vi "CSM - Debug Console 2.vi"() -> ()   [LabVIEW 2017, in "DebugConsole.lvlib"]
doc: "New version of the CSM Debug Console, you can use this tool:\n1. Select an existing CSM instance, open the front panel and block diagram.\n2. Scan the API interfaces of existing CSM instances.\n3. Select an API interface, call synchronously or asynchronously, view the return value.\n4. View the overall program's running log.\n5. Run Scripts."
uses:
  DebugConsole.lvlib
  _Support/Typedef/_CSM_List Module Scope.ctl
  _Support/GlobalEvent/LogFilter/LogFilter.lvclass/LogFilter.ctl
  _Support/Typedef/_CSM_GlobalLog_MSG.ctl
  _Support/Typedef/_CSM_Response Source Message.ctl
  _Support/Typedef/_CSM_GlobalLog_MSG_TYPE.ctl
  _BroadcastDef.ctl
  AdvanceAPI/CSM - Convert Error to Argument.vi
  _Support/GlobalEvent/GEvt-Generate with Rule Check.vi
  _Support/GlobalEvent/Cache-GEvt Filter Object.vi
  _Support/GlobalEvent/Cache-GEvt Refs.vi
  AdvanceAPI/CSM - Keywords.vi
  _Shared/Trim Single-line Text.vi
  AdvanceAPI/CSM - Make String Arguments Safe.vi
  _Support/GlobalEvent/GEvt-Convert Filter Rules - v1.2.vi
  _Support/ChangeFlag/FlagInstance-GEvt Filter.vi
  _Support/ChangeFlag/FlagInstance-GEvt Refs.vi
  _Support/GlobalEvent/LogFilter/SettingVIs/Set Global CSM Filter.vi
  _Support/GlobalEvent/LogFilter/SettingVIs/Set Global LogType Filter.vi
  _Support/GlobalEvent/LogFilter/SettingVIs/Set Global State Filter.vi
  _Support/GlobalEvent/LogFilter/SettingVIs/Set CSM LogType Filter.vi
  _Support/GlobalEvent/LogFilter/SettingVIs/Set CSM State Filter.vi
  _Support/GlobalEvent/LogFilter/SettingVIs/Set Global StateType Filter.vi
  _Support/GlobalEvent/LogFilter/SettingVIs/Set CSM StateType Filter.vi
  _Support/GlobalEvent/LogFilter/SettingVIs/Set Periodic Log Filter.vi
  _Support/GlobalEvent/LogFilter/SettingVIs/Set CSM Broadcast Filter.vi
  _Support/GlobalEvent/LogFilter/SettingVIs/Set Global Broadcast Filter.vi
  _Support/GlobalEvent/LogFilter/SettingVIs/Set Global UserLog Filter.vi
  _Support/GlobalEvent/LogFilter/SettingVIs/Set CSM UserLog Filter.vi
  _Support/ChangeFlag/ChangeFlag-Read.vi
  _csmHelper/API/Create From VI Reference.vi
  _csmHelper/API/Update lvcsm Section in VI Description.vi
  _csmHelper/API/Destroy.vi
  _csmlite/_PassAllowedMessage - MsgList.vi
  _Support/ChangeFlag/ChangeFlagDB.vi
  _Support/GlobalEvent/FGV-GlobalEventRef(lvlibp).vi
  _Support/GlobalEvent/FGV-GlobalEventQueues(lvlibp).vi
  _Support/GlobalEvent/GEvt-Valid Subscribers.vi
  _Support/GlobalEvent/FGV-GEvt Filter Rules(lvlibp).vi
  _Support/GlobalEvent/LogFilter/LogFilter - Check.vi
  HistoryList.vi
  Script-Window.vi
  Module Information.vi
  _Support/GlobalEvent/LogFilter/LogFilter.lvclass
  Communicable State Machine.lvlib
  _csmHelper/API with lvcsm Support/CSM-Helper API with lvcsm Support.lvlib
  _csmHelper/CSM-Helper.lvclass
  _ui/csm-ui-support.lvlib
  _csmlite/_csmlite.lvlib
  _Shared/CSM Shared.lvlib
  _csmlite/_action.ctl
panel:
  in  "Scope":T1
  in  "Refresh CSMs Button":bool
  in  "CSM":string(combo)
  in  "Write lvcsm in Description":bool
  out "inlvlibp":bool
  in  "RetainWireValues":bool
  in  "Toolbar.Exit":bool
  in  "Toolbar.Open FP":bool
  in  "Toolbar.Open BD":bool
  in  "Refresh lvcsm Cache":bool
  in  "Console":T2(tab)
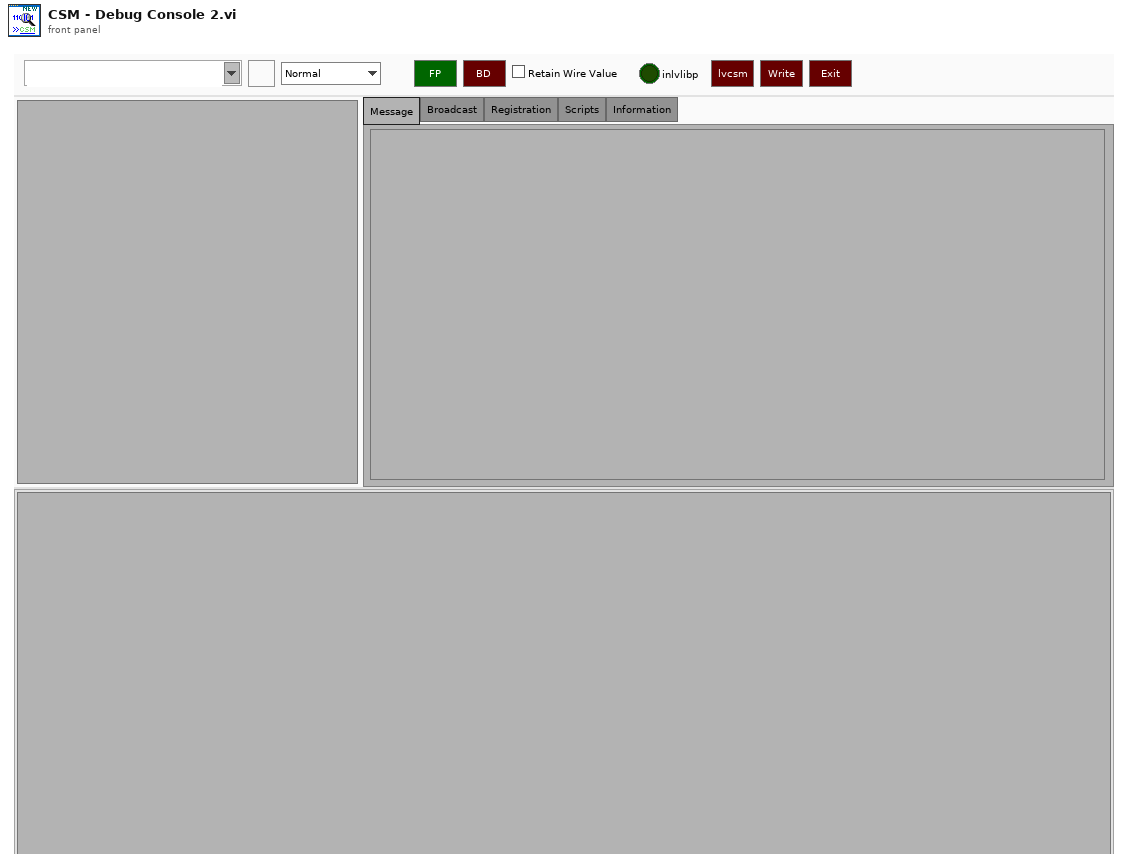
[diagram p1: front panel]
types:
  T1 = typedef "Communicable State Machine.lvlib/_CSM_List Module Scope.ctl" = enum16{"Normal", "System Only", "All"}
  T2 = enum32{"Message", "Broadcast", "Registration", "Scripts", "Information"}
  T3 = cluster{"Left":i32, "Right":i32, "Top":i32, "Bottom":i32}
  T4 = enum32{"Invalid", "Standard", "Closed", "Hidden", "Minimized", "Maximized"}
  T5 = enum32{"invalid app kind", "Development System", "Run Time System", "Student Edition", "Embedded LabVIEW", "Evaluation", "Custom"}
  T6 = typedef "DebugConsole.lvlib/_BroadcastDef.ctl" = enum16{"<no action>", "Macro: Exit", "CSM: Module List Changed", "CSM: Scripts Changed", "CSM: Registration Changed", "CSM: Module Selected", "CSM: Message Excuted", "CSM: Broadcast Excuted", "CSM: Registration Action Excuted", "UI: Try to Change Command"}
  T7 = typedef "_csmlite.lvlib/_action.ctl" = enum16{"Obtain", "Destroy", "Broadcast", "Post", "List"}
  T8 = cluster{"Shift":bool, "Ctrl":bool, "Alt":bool, "Cmd":bool, "Opt":bool}
  T9 = cluster{"Core":cluster{"Current VI Reference":refnum<vi>, "Close Panel on Exit?":bool}, "CSM Global Log Event":refnum<user-event>, "MessageList":string[], "Toobar.advance":refnum<vi>[], "ConsoleUI":refnum<vi>[]}
  T10 = cluster{"Current VI Reference":refnum<vi>, "Close Panel on Exit?":bool}
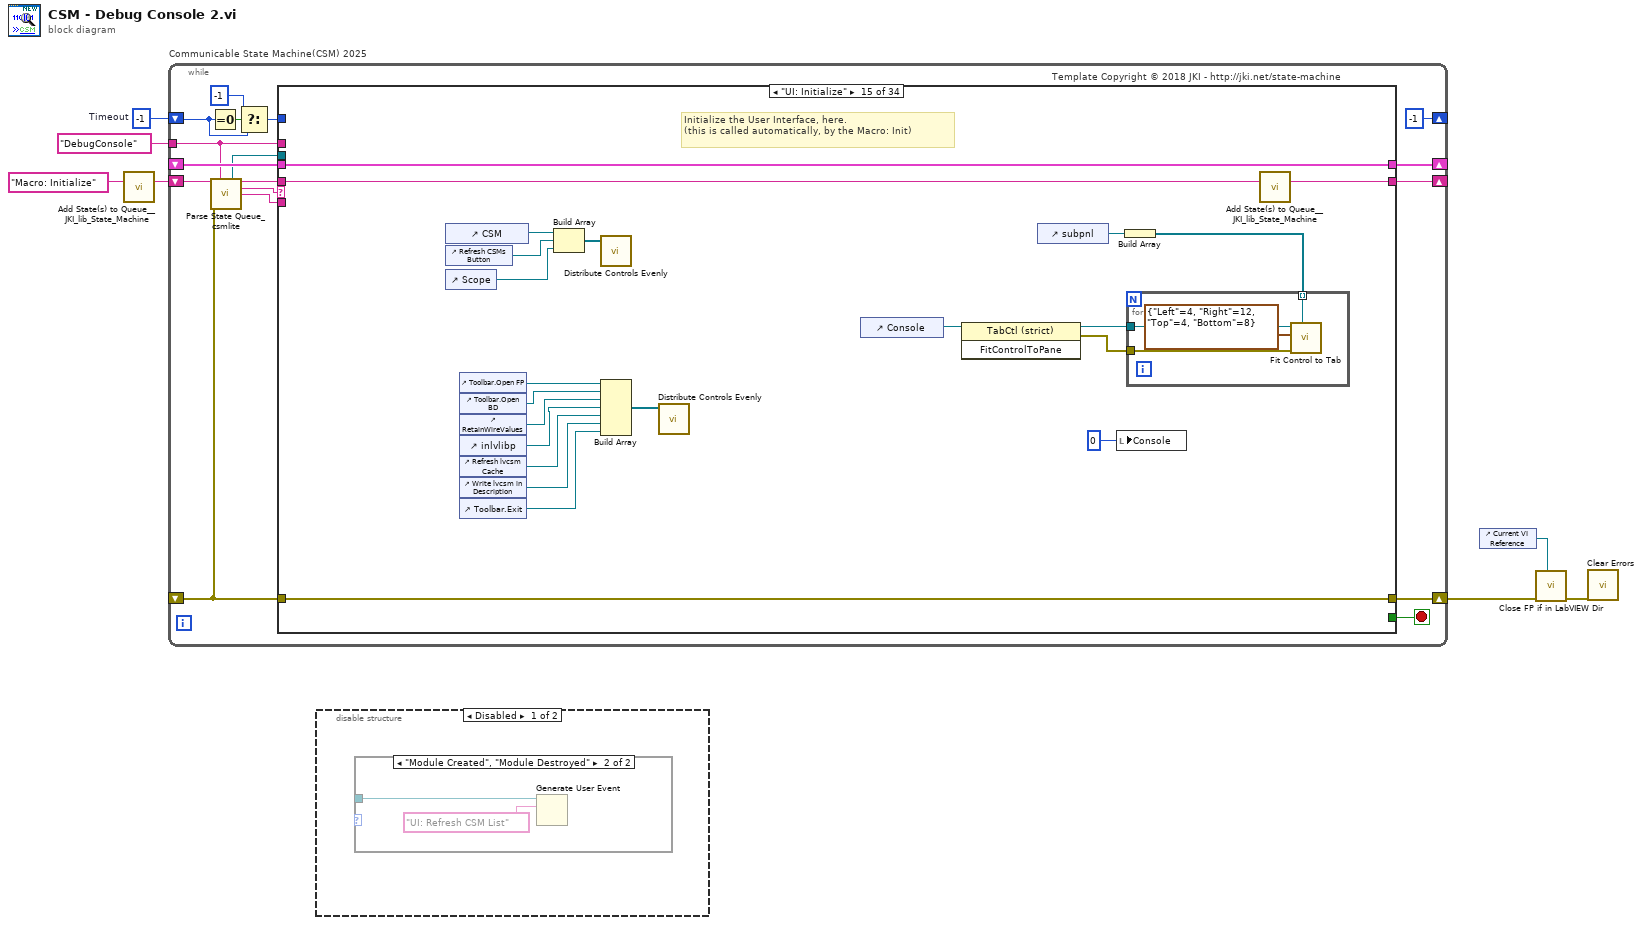
[diagram p0: block diagram]
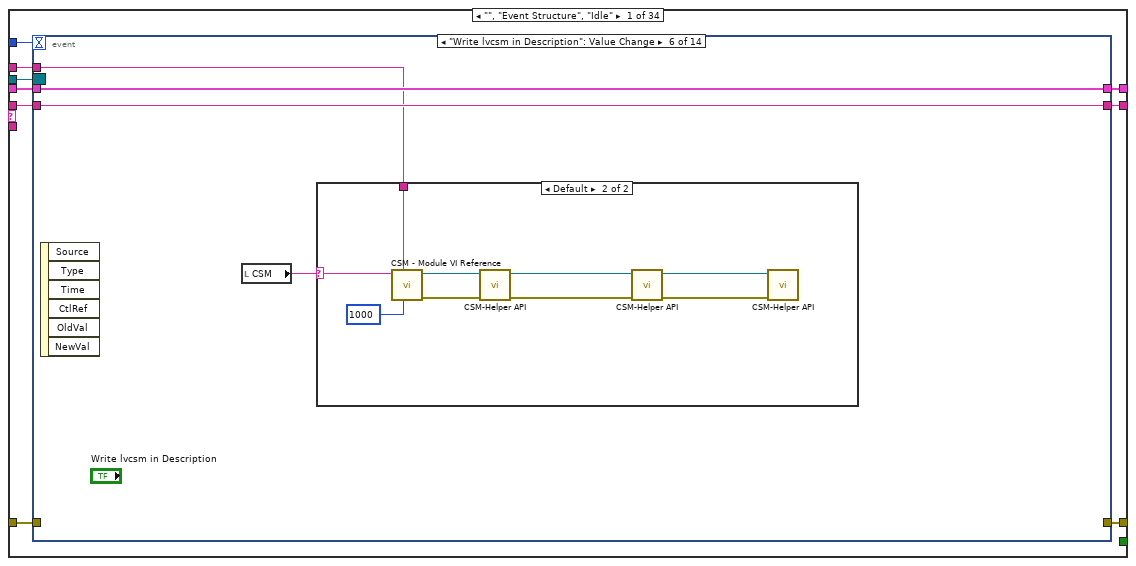
[diagram p4: hidden frame]
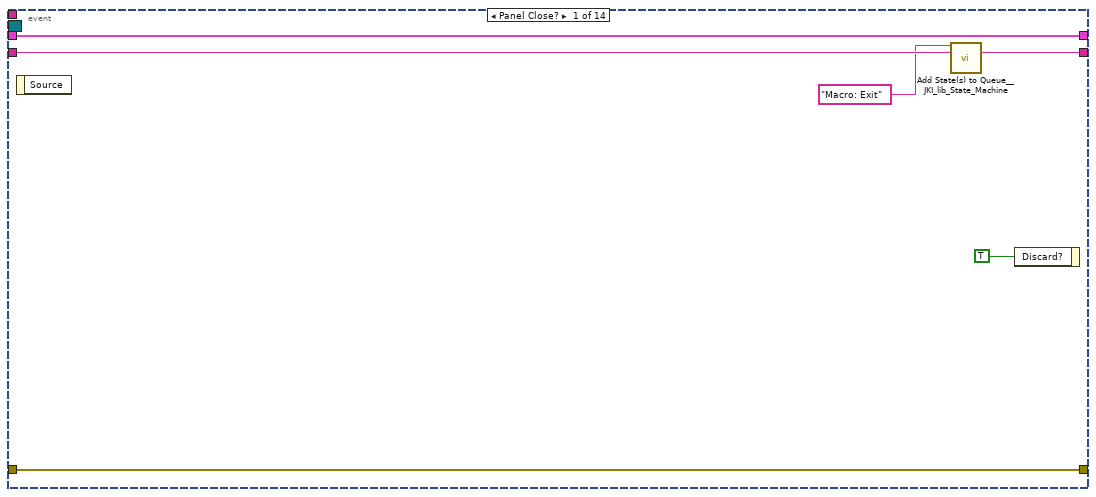
[diagram p5: hidden frame]
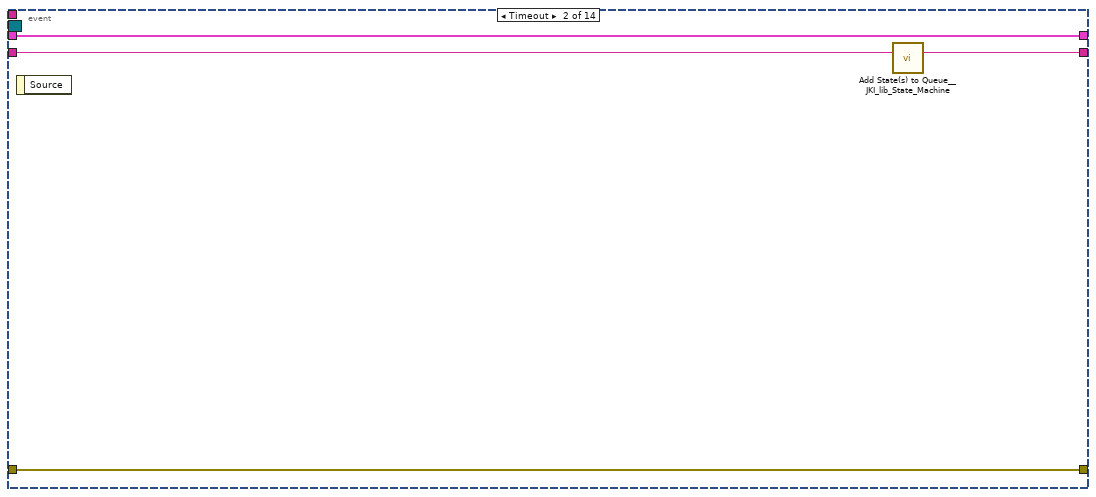
[diagram p6: hidden frame]
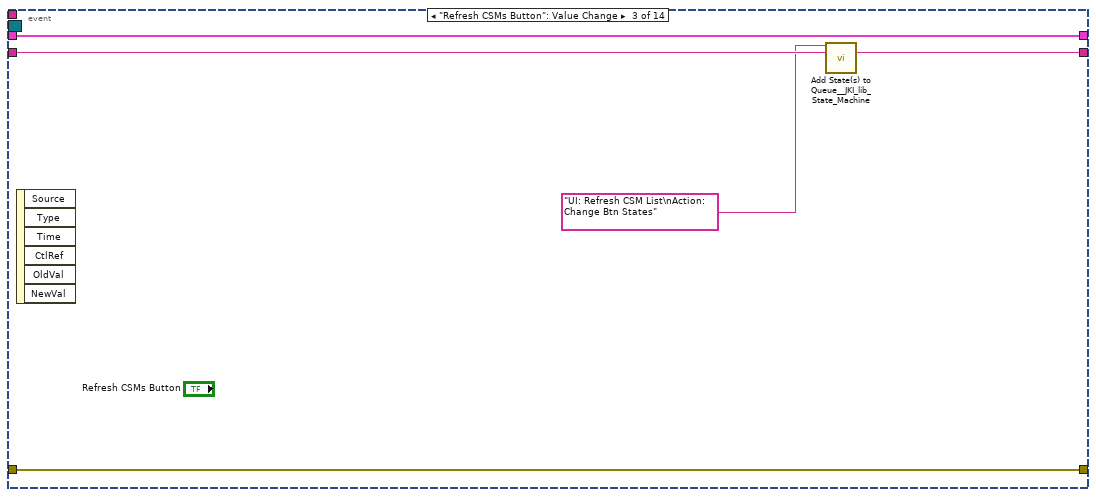
[diagram p7: hidden frame]
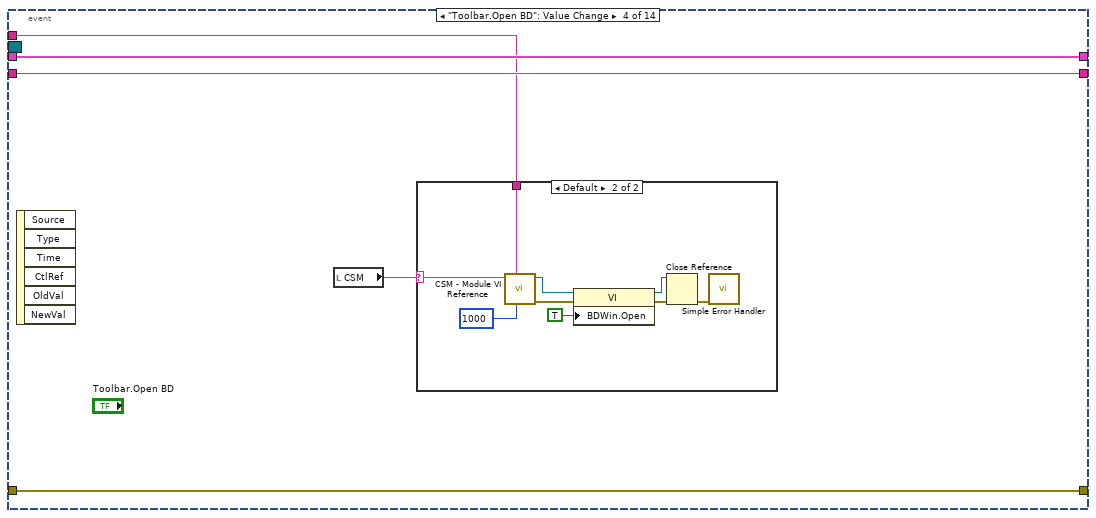
[diagram p8: hidden frame]
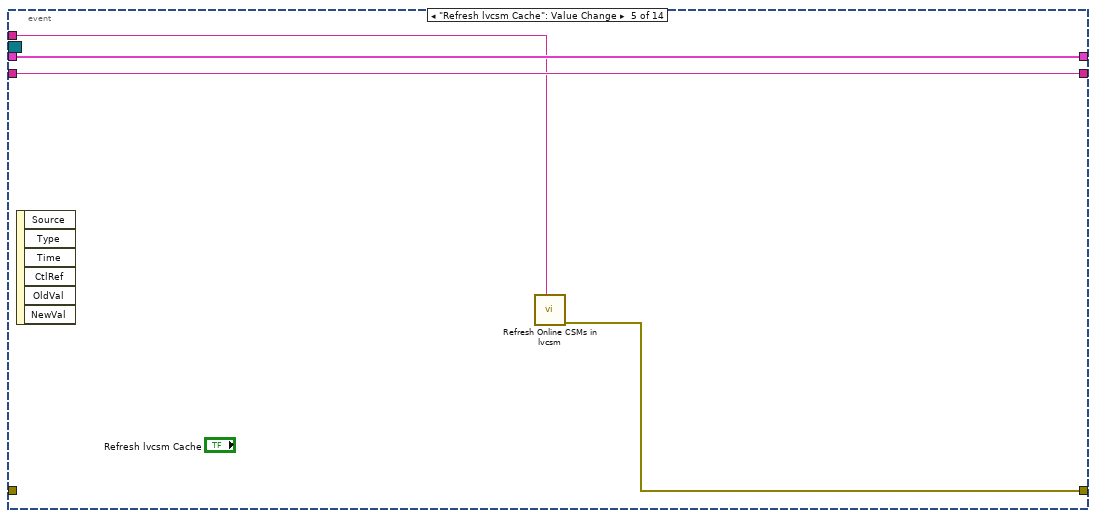
[diagram p10: hidden frame]
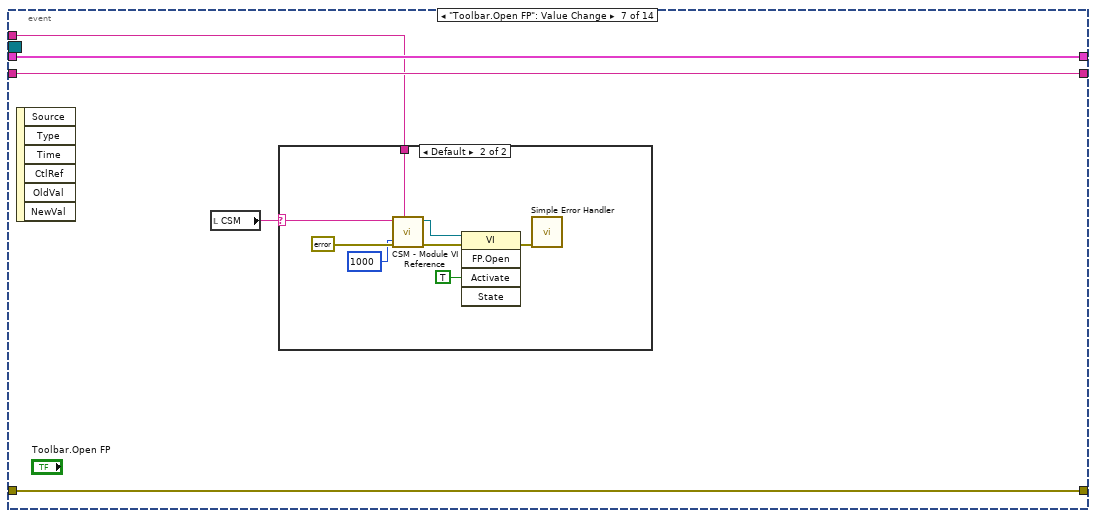
[diagram p12: hidden frame]
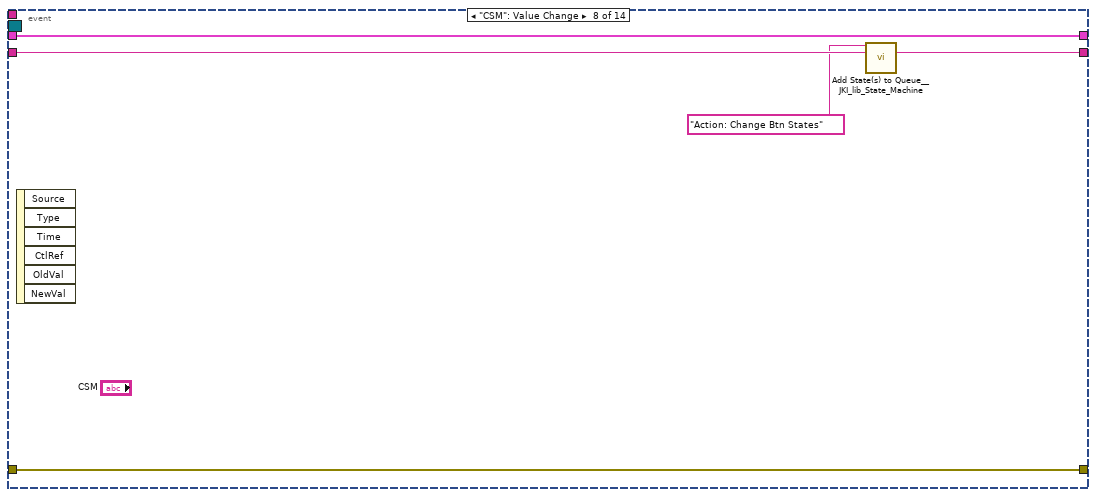
[diagram p14: hidden frame]
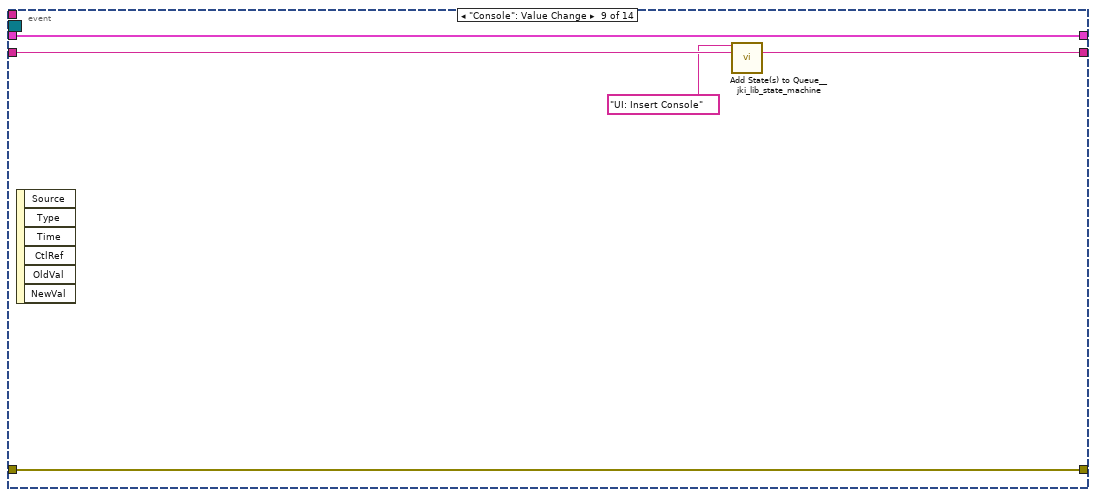
[diagram p15: hidden frame]
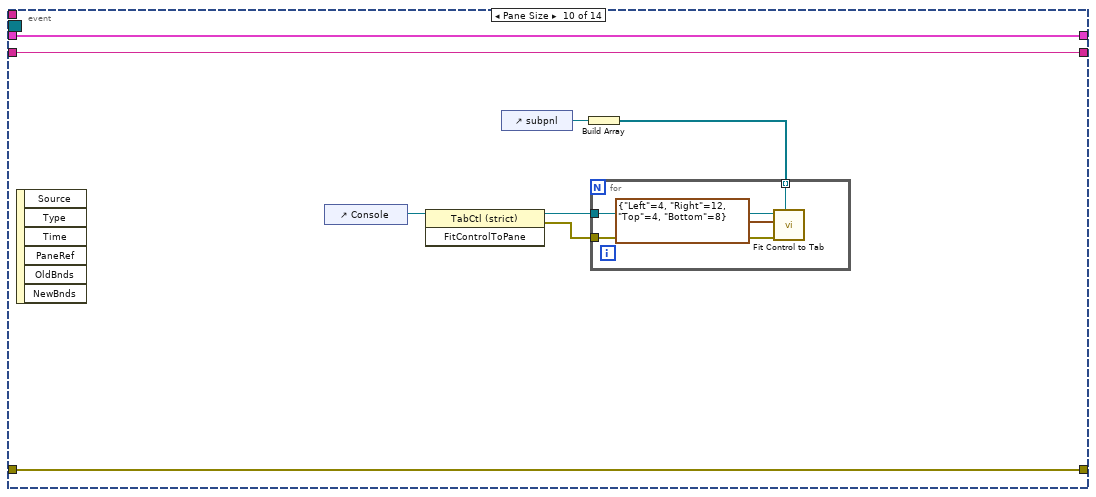
[diagram p16: hidden frame]
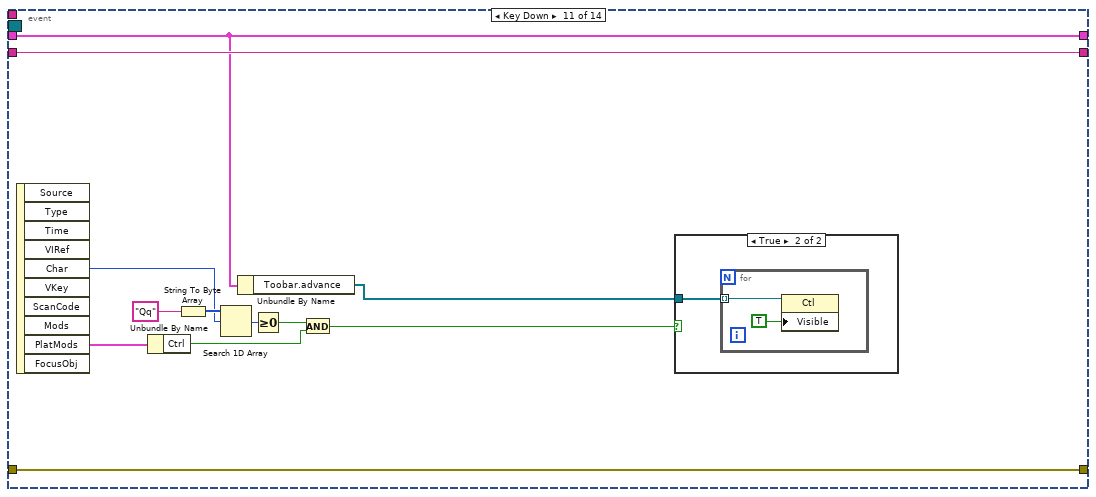
[diagram p17: hidden frame]
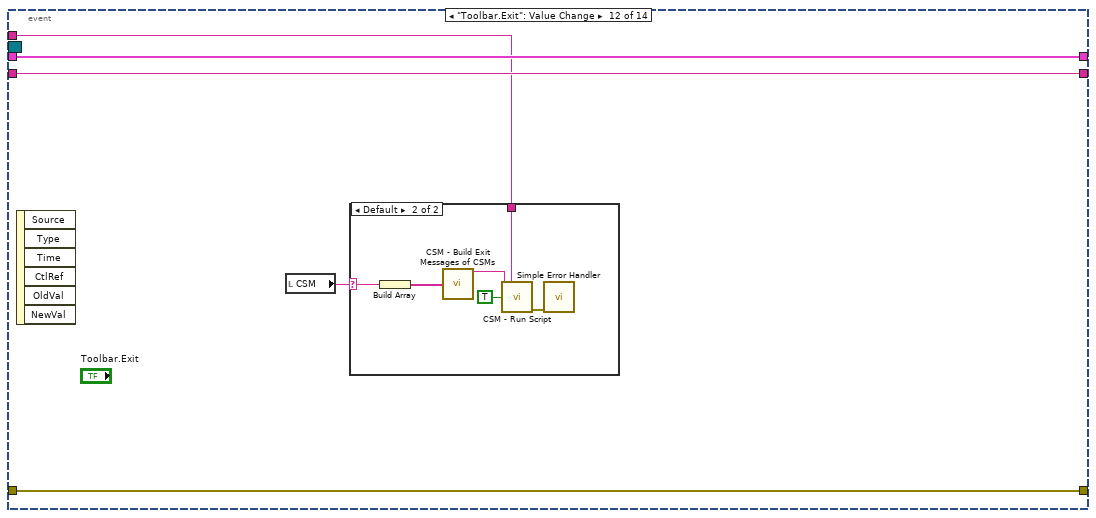
[diagram p19: hidden frame]
diagram:
  w5 = -1  # Timeout
  n1 = call <vilib>:"Add State(s) to Queue__JKI_lib_State_Machine.vi"("State(s) in (\"\")"="Macro: Initialize") -> ("States Out"=w6:string)  [unwired: 14 in]
  n2 = while "Communicable State Machine(CSM) 2025" {
    shift-right: [w17] -> _
    shift-left: _ -> [w16]
    shift-right: [w20] -> w2
    shift-left: _ -> [w15]
    shift-right: [w19] -> _
    shift-left: w6 -> [w21]
    tunnel: "DebugConsole" -> [w9]
    shift-right: [-1 ("Timeout")] -> _
    shift-left: w5 -> [w12]
    stop <- w18 stop-if-true
    # "Template Copyright © 2018 JKI - http://jki.net/state-machine"
    n3 = Equal To 0?(x=w12) -> (x = 0?=w14:bool)
    n4 = call "Parse State Queue_csmlite.vi"("State Queue"=w21, "Current Module(\"\" to generate an ID)"=w9, "Error In (no error)"=w15) -> ("Event Registration Refnum"=w8:refnum<event-registration>, "Remaining States"=w23:string, "Current State"=w24:string, "Arguments"=w22:string)  [unwired: 9 in]
    n5 = Select(t=-1 ("Timeout"), s=w14, f=w12) -> (s? t:f=w11:i32)
    n6 = case shown="\"UI: Initialize\"" w24 {
      selector: w24 -> [_ _ w171 _ _ _ _ _ _ _ _ _ _ _ _ _ _ _ _ _ _ _ _ _ _ _ _ _ _ _ _ _ _ _]
      tunnel: w23 -> [w33 w170 w175 w194 w201 w206 w210 w219 w226 w229 w231 w241 w256 w260 w282 w292 w303 w380 w397 w417 w433 w440 w443 w448 w453 w464 w485 w491 w510 w515 w534 w553 w572 w591]
      tunnel: w22 -> [_ _ _ _ _ _ _ _ _ _ _ w237 _ _ _ w287 w297 _ w394 _ _ _ _ _ _ _ _ _ _ _ _ _ _ _]
      tunnel: w16 -> [w31 w167 w173 w187 w198 w204 w207 _ w225 w228 w230 w239 w251 w257 w279 w290 w299 w379 w396 w416 w432 w438 w442 w445 w450 w461 w482 w490 w509 w514 w533 w552 w571 w590]
      tunnel: [w30 w168 w177 w191 errorcluster {"status"=FALSE, "code"=0, "source"=""} ("error out") w203 w208 w216 w227 _ _ w240 w252 w258 w280 w288 w300 w381 w398 w418 w434 w441 w444 w446 w451 w462 w483 w492 w511 w516 w535 w554 w573 w592] -> w20
      tunnel: w15 -> [w29 w168 w176 w191 w197 w203 w208 w216 w227 _ _ w240 w253 w258 w280 w289 w301 w381 w398 w418 w434 w441 w444 w446 w451 w462 w483 w492 w511 w516 w535 w554 w573 w592]
      tunnel: [w32 w169 w174 w193 w200 w205 w209 w218 w226 w229 w231 w241 w255 w259 w281 w291 w302 w380 w397 w417 w433 w440 w443 w447 w452 w463 w484 w491 w510 w515 w534 w553 w572 w591] -> w19
      tunnel: [_ _ _ _ _ TRUE _ _ _ _ _ _ _ _ _ _ _ _ _ _ _ _ _ _ _ _ _ _ _ _ _ _ _ _] -> w18
      tunnel: [w28 w167 w173 w192 w198 w204 w207 w217 w222 w228 w230 w233 w251 w257 w279 w290 w299 w379 w396 w416 w432 w438 w442 w445 w450 w461 w482 w490 w509 w513 w532 w551 w570 w589] -> w17
      tunnel: w11 -> [w27 _ _ _ _ _ _ _ _ _ _ _ _ _ _ _ _ _ _ _ _ _ _ _ _ _ _ _ _ _ _ _ _ _]
      tunnel: w9 -> [w26 _ _ _ w195 _ _ _ _ _ _ _ _ _ _ _ _ _ _ w405 w421 _ _ _ _ w454 _ w488 w507 w512 w531 w550 w569 w588]
      tunnel: w8 -> [w25 _ _ _ _ _ _ _ _ _ _ _ _ _ _ _ _ _ _ _ _ _ _ _ _ _ _ _ _ _ _ _ _ _]
      frame "", "Event Structure", "Idle" {
        n7 = event shown="[5] \"Write lvcsm in Description\": Value Change" {
          selector: w25 -> [_ _ _ _ _ _ _ _ _ _ _ _ _ _]
          dyn-events: _ -> [_ _ _ _ _ _ _ _ _ _ _ _ _ _]
          timeout: w27 -> [_ _ _ _ _ _ _ _ _ _ _ _ _ _]
          tunnel: w33 -> [w39 w43 w46 w53 w66 w70 w84 w94 w99 w110 w126 w134 w148 w163]
          tunnel: [w38 w42 w45 w53 w66 w70 w84 w95 w100 w110 w126 w134 w148 w164] -> w32
          tunnel: w31 -> [w36 w40 w47 w52 w65 w69 w83 w96 w101 w108 w115 w133 w146 w165]
          tunnel: [w37 w41 w48 w50 w63 _ w81 w97 w102 w109 w125 w132 w147 w166] -> w30
          tunnel: w29 -> [w37 w41 w48 w50 _ _ w81 w97 w102 w109 w125 w132 w147 w166]
          tunnel: [w36 w40 w47 w52 w65 w69 w83 w96 w101 w108 w115 w133 w146 w165] -> w28
          tunnel: w26 -> [_ _ _ w49 w64 w67 w80 _ _ _ _ w130 w144 _]
          event Panel Close? {
            n8 = event-data() -> ()  [unwired: 1 in, 1 out]
            n9 = call <vilib>:"Add State(s) to Queue__JKI_lib_State_Machine.vi"("State(s) in Front (\"\")"="Macro: Exit", "State(s) in (\"\")"=w39) -> ("States Out"=w38:string)  [unwired: 13 in]
            n10 = event-data("Discard?"=TRUE) -> ()  [unwired: 1 in, 1 out]
          }
          event Timeout {
            n11 = event-data() -> ()  [unwired: 1 in, 1 out]
            n12 = call <vilib>:"Add State(s) to Queue__JKI_lib_State_Machine.vi"("State(s) in (\"\")"=w43) -> ("States Out"=w42:string)  [unwired: 14 in]
          }
          event "Refresh CSMs Button": Value Change {
            n13 = event-data() -> ()  [unwired: 1 in, 6 out]
            n14 = call <vilib>:"Add State(s) to Queue__JKI_lib_State_Machine.vi"("State(s) in Front (\"\")"="UI: Refresh CSM List\nAction: Change Btn States" ("State(s) in Front (\"\")"), "State(s) in (\"\")"=w46) -> ("States Out"=w45:string)  [unwired: 13 in]
          }
          event "Toolbar.Open BD": Value Change {
            n15 = event-data() -> ()  [unwired: 1 in, 6 out]
            n16 = local read "CSM"() -> (w51:string)
            n17 = case shown="Default" w51 {
              selector: w51 -> [_ w61]
              tunnel: w49 -> [_ w60]
              frame "" {
              }
              frame Default {
                n18 = call "CSM - Module VI Reference.vi"("Response Timeout (-2 Using Global Settings)"=1000 ("Response Timeout(5000 ms)"), "Current Module (\"\" to Generate an ID)"=w60, "CSM Name"=w61) -> ("error out"=w54:errorcluster, "CSM Module VIRef"=w59:refnum<vi>)  [unwired: 7 in]
                n19 = property class="VI"(reference=w59, error in=w54, "BDWin.Open"=TRUE ("Block Diagram Window:Open")) -> (reference out=w57:refnum<vi>, error out=w56:errorcluster)
                n20 = Close Reference(reference=w57, error in (no error)=w56) -> (error out=w62:errorcluster)
                n21 = call <vilib>:"Simple Error Handler.vi"("error in (no error)"=w62) -> ()  [unwired: 4 in, 5 out]
              }
            }
          }
          event "Refresh lvcsm Cache": Value Change {
            n22 = event-data() -> ()  [unwired: 1 in, 6 out]
            n23 = call "Refresh Online CSMs in lvcsm.vi"("Caller"=w64) -> ("error out"=w63:errorcluster)  [unwired: 9 in, 1 out]
          }
          event "Write lvcsm in Description": Value Change {
            n24 = event-data() -> ()  [unwired: 1 in, 6 out]
            n25 = local read "CSM"() -> (w68:string)
            n26 = case shown="Default" w68 {
              selector: w68 -> [_ w75]
              tunnel: w67 -> [_ w71]
              frame "" {
              }
              frame Default {
                n27 = call "CSM - Module VI Reference.vi"("Response Timeout (-2 Using Global Settings)"=1000 ("Response Timeout(5000 ms)"), "Current Module (\"\" to Generate an ID)"=w71, "CSM Name"=w75) -> ("error out"=w73:errorcluster, "CSM Module VIRef"=w72:refnum<vi>)  [unwired: 7 in]
                n28 = call-poly "CSM-Helper API.vi"("error in (no error)"=w73, "VI"=w72) -> ("error out"=w79:errorcluster, "CSM-Helper.lvclass"=w78:refnum<class "CSM-Helper.lvclass">)  [unwired: 8 in]
                n29 = call-poly "CSM-Helper API.vi"("error in (no error)"=w79, "CSM-Helper in"=w78) -> ("error out"=w77:errorcluster, "CSM-Helper out"=w76:refnum<class "CSM-Helper.lvclass">)  [unwired: 8 in]
                n30 = call-poly "CSM-Helper API.vi"("error in (no error)"=w77, "CSM-Helper in"=w76) -> ()  [unwired: 8 in, 2 out]
              }
            }
          }
          event "Toolbar.Open FP": Value Change {
            n31 = event-data() -> ()  [unwired: 1 in, 6 out]
            n32 = local read "CSM"() -> (w82:string)
            n33 = case shown="Default" w82 {
              selector: w82 -> [_ w92]
              tunnel: w80 -> [_ w90]
              frame "" {
              }
              frame Default {
                n34 = call "CSM - Module VI Reference.vi"("Response Timeout (-2 Using Global Settings)"=1000 ("Response Timeout(5000 ms)"), "Current Module (\"\" to Generate an ID)"=w90, "error in (no error)"=errorcluster {"status"=FALSE, "code"=0, "source"=""}, "CSM Name"=w92) -> ("error out"=w86:errorcluster, "CSM Module VIRef"=w87:refnum<vi>)  [unwired: 6 in]
                n35 = invoke on="Invoke Node" class="VI" method="FP.Open"(reference=w87, error in=w86, "Activate"=TRUE ("Activate?")) -> (error out=w91:errorcluster)  [unwired: 2 in, 4 out]
                n36 = call <vilib>:"Simple Error Handler.vi"("error in (no error)"=w91) -> ()  [unwired: 4 in, 5 out]
              }
            }
          }
          event "CSM": Value Change {
            n37 = event-data() -> ()  [unwired: 1 in, 6 out]
            n38 = call <vilib>:"Add State(s) to Queue__JKI_lib_State_Machine.vi"("State(s) in Front (\"\")"="Action: Change Btn States" ("State(s) in Front (\"\")"), "State(s) in (\"\")"=w94) -> ("States Out"=w95:string)  [unwired: 13 in]
          }
          event "Console": Value Change {
            n39 = event-data() -> ()  [unwired: 1 in, 6 out]
            n40 = call <vilib>:"Add State(s) to Queue__jki_lib_state_machine.vi"("State(s) in Front (\"\")"="UI: Insert Console" ("State(s) in Front (\"\")"), "State(s) in (\"\")"=w99) -> ("States Out"=w100:string)  [unwired: 13 in]
          }
          event Pane Size {
            n41 = event-data() -> ()  [unwired: 1 in, 6 out]
            n42 = control-ref of="Console"() -> (w105:refnum<vi>)
            n43 = invoke class="TabCtl (strict)" method="FitControlToPane"(reference=w105) -> (reference out=w107:refnum<vi>, error out=w106:errorcluster)  [unwired: 2 in, 1 out]
            n44 = control-ref of="subpnl"() -> (w104:refnum<vi>)
            n45 = Build Array(w104) -> (w103:refnum<vi>[])
            n46 = for {
              tunnel: w107 -> [w114]
              tunnel: w103 -> [w113] mode=indexing
              tunnel: w106 -> [w112]
              n47 = call "Fit Control to Tab.vi"("Control"=w113, "error in (no error)"=w112, "Margin"=T3 {"Left"=4, "Right"=12, "Top"=4, "Bottom"=8}, "TabRef"=w114) -> ()  [unwired: 3 in, 3 out]
            }
          }
          event Key Down {
            n48 = event-data() -> ("Char"=w116:i16, "PlatMods"=w117:T8)  [unwired: 1 in, 8 out]
            n49 = Unbundle By Name(w117) -> ("Ctrl"=w120:bool)
            n50 = String To Byte Array(string="Qq") -> (unsigned byte array=w122:u8[])
            n51 = Search 1D Array(1D array=w122, element=w116) -> (index of element=w123:i32)  [unwired: 1 in]
            n52 = Unbundle By Name(w115) -> ("Toobar.advance"=w118:refnum<vi>[])
            n53 = Greater Or Equal To 0?(x=w123) -> (x >= 0?=w124:bool)
            n54 = And(x=w124, y=w120) -> (x .and. y?=w119:bool)
            n55 = case shown="True" w119 {
              tunnel: w118 -> [_ w127]
              frame False {
              }
              frame True {
                n56 = for {
                  tunnel: w127 -> [w129] mode=indexing
                  n57 = property class="Ctl"(reference=w129, "Visible"=TRUE) -> ()  [unwired: 1 in, 2 out]
                }
              }
            }
          }
          event "Toolbar.Exit": Value Change {
            n58 = event-data() -> ()  [unwired: 1 in, 6 out]
            n59 = local read "CSM"() -> (w131:string)
            n60 = case shown="Default" w131 {
              selector: w131 -> [_ w137]
              tunnel: w130 -> [_ w140]
              frame "" {
              }
              frame Default {
                n61 = Build Array(w137) -> (w136:string[])
                n62 = call "CSM - Build Exit Messages of CSMs.vi"("CSMs"=w136) -> ("States"=w138:string)  [unwired: 14 in]
                n63 = call "CSM - Run Script.vi"("CSM Scripts"=w138, "Current Module (\"\" to Generate an ID)"=w140, "Continue If Error? (F)"=TRUE) -> ("error out"=w139:errorcluster)  [unwired: 10 in, 2 out]
                n64 = call <vilib>:"Simple Error Handler.vi"("error in (no error)"=w139) -> ()  [unwired: 4 in, 5 out]
              }
            }
          }
          event "RetainWireValues": Value Change {
            n65 = event-data() -> ("CtlRef"=w142:refnum<vi>, "OldVal"=w141:bool, "NewVal"=w143:bool)  [unwired: 1 in, 3 out]
            n66 = local read "CSM"() -> (w145:string)
            n67 = case shown="Default" w145 {
              selector: w145 -> [_ w154]
              tunnel: w144 -> [_ w153]
              tunnel: w143 -> [_ w152]
              tunnel: w142 -> [_ w150]
              tunnel: w141 -> [_ w149]
              frame "" {
              }
              frame Default {
                n68 = call "CSM - Module VI Reference.vi"("Current Module (\"\" to Generate an ID)"=w153, "CSM Name"=w154) -> ("error out"=w156:errorcluster, "CSM Module VIRef"=w155:refnum<vi>)  [unwired: 8 in]
                n69 = property class="VI"(reference=w155, error in=w156, "Exec.PostExecutionProbes"=w152) -> (error out=w151:errorcluster)  [unwired: 1 out]
                n70 = case shown="Error" w151 {
                  selector: w151 -> [_ w157]
                  tunnel: w150 -> [_ w159]
                  tunnel: w149 -> [_ w158]
                  frame No Error {
                  }
                  frame Error {
                    n71 = call <vilib>:"Simple Error Handler.vi"("error in (no error)"=w157) -> ()  [unwired: 4 in, 5 out]
                    n72 = property class="Bool (strict)"(reference=w159, "Value"=w158) -> ()  [unwired: 1 in, 2 out]
                  }
                }
              }
            }
          }
          event User Event {
            n73 = event-data() -> ("Message Event"=w162:string)  [unwired: 1 in]
            n74 = call-poly "Pass Allowed Message.vi"("Allowed Message"=string[] ["Macro: Exit", "CSM: Module List Changed", "UI: Try to Change Command"], "JKISM External Event"=w162) -> ("States"=w161:string)  [unwired: 7 in]
            n75 = call <vilib>:"Add State(s) to Queue__JKI_lib_State_Machine.vi"("State(s) in Front (\"\")"=w161, "State(s) in (\"\")"=w163) -> ("States Out"=w164:string)  [unwired: 13 in]
          }
        }
      }
      frame "---------- Core ----------" {
        # "Do not put any code in this frame.\n(it is a separator no-op)"
        n76 = call <vilib>:"Add State(s) to Queue__JKI_lib_State_Machine.vi"("State(s) in (\"\")"=w170) -> ("States Out"=w169:string)  [unwired: 14 in]
      }
      frame Default {
        w180 = 42 items=["No error", "Argument error", "Memory is full", "Out of zone", "End of file", "File already open", "Generic file I/O error", "File not found", "File permission error", "Disk is full", "Duplicate path", "Too many files open", "System feature not enabled", "Resource file not found", "Cannot add resource", "Resource not found", "Image not found", "Image memory error", "Pen does not exist", "Config type invalid", "Config token not found", "Config parse error", "Config memory error", "Bad external code format", "Bad external code offset", "External code not present", "Null window", "Destroy window error", "Null menu", "Print aborted", "Bad print record", "Print driver error", "Windows error during printing", "Memory error during printing", "Print dialog error", "Generic print error", "Invalid device refnum", "Device not found", "Device parameter error", "Device unit error", "Cannot open device", "Device call aborted", "Generic error", "Cancelled by user", "Object ID too low", "Object ID too high", "Object not in heap", "Unknown heap", "Unknown object (invalid DefProc)", "Unknown object (DefProc not in table)", "Message out of range", "Invalid (null) method", "Unknown message", "Manager call not supported", "Bad address", "Network operation in progress", "Network operation timed out", "Connection is busy", "Network attribute not supported", "Network error", "Address in use", "System out of memory", "Connection aborted", "Connection refused", "Not connected", "Already connected", "Connection closed", "Initialization error (interapplication manager)", "Bad occurrence", "Wait on unbound occurrence handler", "Occurrence queue overflow", "Datalog type conflict", "Unused", "Unrecognized type (interapplication manager)", "Memory corrupt", "Failed to make temporary DLL", "Old CIN version", "Drag socket not found", "Failed to load drop-object", "Failed to register OLE object", "Failed to release OLE object", "Format specifier type mismatch", "Unknown format specifier", "Too few format specifiers", "Too many format specifiers", "Scan failed", "Newer CIN version", "Error converting to variant", "Runtime menu error", "Password tampered", "Variant attribute not found", "Incompatible variant data type", "Event data is not available", "Event Store is not present", "Occurrence is not found", "Event Queue is not created", "Event info is not available", "Refnum passed is NULL", "Error retrieving Class GUID", "Error retrieving CoClass GUID", "Error retrieving TypeLib GUID.", "Bad built application magic bytes.", "Specific driver is different from the specific driver associated with the Logical Name.", "There is no session opened to the class driver.", "Max Error", "MAX - Error with config objects", "MAX - Error loading configuration", "MAX - Group not supported"]
        # "Current State"
        # "Do not delete, rename, or modify this frame.\n(this is used to capture unhandled states and typos)"
        # "Handle mistyped state name (developer tool)"
        n77 = Format Into String(format string="Software Exception: Unhandled State \"%s\"." ("message"), error in=w176, w171) -> (resulting string=w179:string, error out=w178:errorcluster)  [unwired: 1 in]
        n78 = call <vilib>:"Error Cluster From Error Code.vi"("show call chain? (False)"=TRUE, "error in (no error)"=w178, "error message (\"\")"=w179, "error code (0)"=w180) -> ("error out"=w177:errorcluster)  [unwired: 5 in]
        n79 = call <vilib>:"Add State(s) to Queue__JKI_lib_State_Machine.vi"("State(s) in (\"\")"=w175) -> ("States Out"=w174:string)  [unwired: 14 in]
      }
      frame "Initialize Core Data" {
        # "Do not delete, rename, or modify this frame.\n(this is used to determine panel behavior on exit)"
        # "originally closed?"
        # "exe?"
        # "If panel starts closed or is an EXE, then close it when we exit"
        n80 = property class="VI"() -> ("FP.State"=w184:T4)  [unwired: 2 in, 2 out]
        n81 = property class="App"() -> ("App.Kind"=w190:T5)  [unwired: 2 in, 2 out]
        n82 = control-ref of="Current VI Reference"() -> (w185:refnum<vi>)
        n83 = Equal?(x=w184, y=T4."Closed" ("Front Panel Window:State")) -> (x = y?=w182:bool)
        n84 = Equal?(x=w190, y=T5."Run Time System" ("Application:Kind")) -> (x = y?=w188:bool)
        n85 = Or(x=w182, y=w188) -> (x .or. y?=w186:bool)
        n86 = Bundle By Name(cluster=w187, "Core.Current VI Reference"=w185, "Core.Close Panel on Exit?"=w186) -> (w192:T9)
        n87 = call <vilib>:"Add State(s) to Queue__JKI_lib_State_Machine.vi"("State(s) in (\"\")"=w194) -> ("States Out"=w193:string)  [unwired: 14 in]
      }
      frame "Error Handler" {
        # "Unhandled Error -- Display it"
        # "Handle any errors here.\nYou can also output any states to clean-up after errors occur"
        # "Clear error"
        n88 = call "CSM - Global Log Error Handler.vi"("Place (\"\" to Use VI's Name)"=w195, "Error In"=w197) -> ()  [unwired: 9 in, 1 out]
        n89 = call <vilib>:"Add State(s) to Queue__JKI_lib_State_Machine.vi"("State(s) in Front (\"\")"="/* Post Error States", "State(s) in (\"\")"=w201) -> ("States Out"=w200:string)  [unwired: 13 in]
      }
      frame "Exit" {
        # "Do not put any code in this frame.\n(No errors that occur here will be handled.)"
        n90 = call <vilib>:"Add State(s) to Queue__JKI_lib_State_Machine.vi"("State(s) in (\"\")"=w206) -> ("States Out"=w205:string)  [unwired: 14 in]
      }
      frame "---------- Data ----------" {
        # "Do not put any code in this frame.\n(It is a separator no-op. You can make a copy of this frame to create a new Data frame)"
        n91 = call <vilib>:"Add State(s) to Queue__JKI_lib_State_Machine.vi"("State(s) in (\"\")"=w210) -> ("States Out"=w209:string)  [unwired: 14 in]
      }
      frame "Data: Initialize" {
        w211 = refnum<vi>[] []  # ConsoleUI
        w212 = refnum<vi>[] []  # Toobar.advance
        w213 = string[] []  # MessageList
        w214 = refnum<user-event> refnum  # CSM Global Log Event
        w215 = T10 {"Current VI Reference"=refnum, "Close Panel on Exit?"=FALSE}  # Core
        # "Initialize the shift-register data, here.\n(data names are defined by what you wire into the bundle function)"
        n92 = Bundle("Core"=w215, "CSM Global Log Event"=w214, "MessageList"=w213, "Toobar.advance"=w212, "ConsoleUI"=w211) -> (w217:T9)  [unwired: 1 in]
        n93 = call <vilib>:"Add State(s) to Queue__JKI_lib_State_Machine.vi"("State(s) in (\"\")"=w219) -> ("States Out"=w218:string)  [unwired: 14 in]
      }
      frame "Data: Initialize References" {
        n94 = control-ref of="Toolbar.Open FP"() -> (w224:refnum<vi>)
        n95 = control-ref of="Toolbar.Open BD"() -> (w223:refnum<vi>)
        n96 = control-ref of="Refresh lvcsm Cache"() -> (w220:refnum<vi>)
        n97 = Build Array(w224, w223, w220) -> (w221:refnum<vi>[])
        n98 = Bundle By Name(cluster=w225, "Toobar.advance"=w221) -> (w222:T9)
      }
      frame "Data: Load Arguments Config File" {
      }
      frame "Data: Save Arguments Config File" {
      }
      frame "Data: Update Message List" {
        n99 = Unbundle By Name(w239) -> ("MessageList"=w238:string[])
        n100 = call "CSM - Revert Arguments-Safe String.vi"("Safe Argument String"=w237) -> ("Origin Argument String"=w236:string)  [unwired: 8 in]
        n101 = Build Array (concatenate)(w236, w238) -> (w235:string[])
        n102 = for {
          tunnel: w235 -> [w245] mode=indexing
          shift-right: [w244] -> w232
          shift-left: string[] [] -> [w243]
          i -> [w242]
          n103 = Search 1D Array(1D array=w243, element=w245) -> (index of element=w246:i32)  [unwired: 1 in]
          n104 = case shown="-1" w246 {
            tunnel: w245 -> [_ w250]
            tunnel: [w247 w248] -> w244
            tunnel: w243 -> [w247 w249]
            tunnel: w242 -> [_ _]
            frame Default {
            }
            frame -1 {
              n105 = Build Array (concatenate)(w249, w250) -> (w248:string[])
            }
          }
        }
        n106 = Bundle By Name(cluster=w239, "MessageList"=w232) -> (w233:T9)
      }
      frame "Data: Cleanup" {
        # "Cleanup any data and references, here.\n(this is called automatically, by the Macro: Exit)"
        n107 = Unbundle By Name(w251) -> ("Core.Current VI Reference"=w254:refnum<vi>)
        n108 = Close Reference(reference=w254, error in (no error)=w253) -> (error out=w252:errorcluster)
        n109 = call <vilib>:"Add State(s) to Queue__JKI_lib_State_Machine.vi"("State(s) in (\"\")"=w256) -> ("States Out"=w255:string)  [unwired: 14 in]
      }
      frame "---------- UI ----------" {
        # "Do not put any code in this frame.\n(It is a separator no-op. You can make a copy of this frame to create a new UI frame)"
        n110 = call <vilib>:"Add State(s) to Queue__JKI_lib_State_Machine.vi"("State(s) in (\"\")"=w260) -> ("States Out"=w259:string)  [unwired: 14 in]
      }
      frame "UI: Initialize" {
        # "Initialize the User Interface, here.\n(this is called automatically, by the Macro: Init)"
        n111 = control-ref of="CSM"() -> (w272:refnum<vi>)
        n112 = control-ref of="Refresh CSMs Button"() -> (w271:refnum<vi>)
        n113 = control-ref of="Scope"() -> (w270:refnum<vi>)
        n114 = control-ref of="Toolbar.Open FP"() -> (w262:refnum<vi>)
        n115 = control-ref of="Toolbar.Open BD"() -> (w263:refnum<vi>)
        n116 = control-ref of="RetainWireValues"() -> (w264:refnum<vi>)
        n117 = control-ref of="inlvlibp"() -> (w265:refnum<vi>)
        n118 = control-ref of="Refresh lvcsm Cache"() -> (w266:refnum<vi>)
        n119 = control-ref of="Write lvcsm in Description"() -> (w267:refnum<vi>)
        n120 = control-ref of="Toolbar.Exit"() -> (w268:refnum<vi>)
        n121 = Build Array(w272, w271, w270) -> (w269:refnum<vi>[])
        n122 = call "Distribute Controls Evenly.vi"("Controls"=w269) -> ()  [unwired: 10 in, 1 out]
        n123 = Build Array(w262, w263, w264, w265, w266, w267, w268) -> (w261:refnum<vi>[])
        n124 = call "Distribute Controls Evenly.vi"("Controls"=w261) -> ()  [unwired: 10 in, 1 out]
        n125 = control-ref of="Console"() -> (w276:refnum<vi>)
        n126 = invoke class="TabCtl (strict)" method="FitControlToPane"(reference=w276) -> (reference out=w278:refnum<vi>, error out=w277:errorcluster)  [unwired: 2 in, 1 out]
        n127 = control-ref of="subpnl"() -> (w275:refnum<vi>)
        n128 = local write "Console"(0) -> ()
        n129 = Build Array(w275) -> (w274:refnum<vi>[])
        n130 = for {
          tunnel: w278 -> [w286]
          tunnel: w274 -> [w285] mode=indexing
          tunnel: w277 -> [w284]
          n131 = call "Fit Control to Tab.vi"("Control"=w285, "error in (no error)"=w284, "Margin"=T3 {"Left"=4, "Right"=12, "Top"=4, "Bottom"=8}, "TabRef"=w286) -> ()  [unwired: 3 in, 3 out]
        }
        n132 = call <vilib>:"Add State(s) to Queue__JKI_lib_State_Machine.vi"("State(s) in (\"\")"=w282) -> ("States Out"=w281:string)  [unwired: 14 in]
      }
      frame "UI: Cursor Set" {
        # "Argument"
        # "Set and Unset Cursor Busy.\n(Usage: \"UI: Cursor Set >> Busy|Idle\")"
        n133 = case shown="\"Idle\", Default" w287 {
          tunnel: w289 -> [w294 w296]
          tunnel: [w293 w295] -> w288
          frame "Idle", Default {
            n134 = call <vilib>:"Unset Busy.vi"("error in (no error)"=w294) -> ("error out"=w293:errorcluster)  [unwired: 10 in]
          }
          frame "Busy" {
            n135 = call <vilib>:"Set Busy.vi"("error in (no error)"=w296) -> ("error out"=w295:errorcluster)  [unwired: 9 in, 1 out]
          }
        }
        n136 = call <vilib>:"Add State(s) to Queue__JKI_lib_State_Machine.vi"("State(s) in (\"\")"=w292) -> ("States Out"=w291:string)  [unwired: 14 in]
      }
      frame "UI: Front Panel State" {
        # "Argument"
        # "Set Front Panel Open or Closed\n(Usage: \"UI: Front Panel State >> Open|Close\")"
        n137 = Unbundle By Name(w299) -> ("Core.Current VI Reference"=w298:refnum<vi>)
        n138 = case shown="\"Minimize\", \"Minimized\"" w297 {
          tunnel: w301 -> [w309 w324 w335 w348 w361]
          tunnel: [w311 w325 w337 w350 w363] -> w300
          tunnel: w298 -> [w310 w322 w336 w349 w362]
          frame "Open", "Standard", Default {
            w304 = T4."Standard" ("State")
            n139 = property class="VI"(reference=w310, error in=w309) -> (reference out=w307:refnum<vi>, error out=w308:errorcluster, "FP.State"=w306:T4)
            n140 = Not Equal?(x=w306, y=w304) -> (x != y?=w305:bool)
            n141 = case shown="True" w305 {
              tunnel: [w315 w317] -> w311
              tunnel: w308 -> [w314 w317]
              tunnel: w307 -> [w313 _]
              tunnel: w304 -> [w312 _]
              frame True {
                n142 = invoke class="VI" method="FP.Open"(reference=w313, error in=w314, "Activate"=TRUE, "State"=w312) -> (error out=w315:errorcluster)  [unwired: 1 in, 4 out]
              }
              frame False {
              }
            }
          }
          frame "Close", "Closed" {
            n143 = property class="VI"(reference=w322, error in=w324) -> (reference out=w321:refnum<vi>, error out=w323:errorcluster, "FP.State"=w319:T4)
            n144 = Not Equal?(x=w319, y=T4."Closed" ("Front Panel Window:State")) -> (x != y?=w318:bool)
            n145 = case shown="True" w318 {
              tunnel: [w326 w329] -> w325
              tunnel: w323 -> [w326 w328]
              tunnel: w321 -> [_ w327]
              frame False {
              }
              frame True {
                n146 = invoke class="VI" method="FP.Close"(reference=w327, error in=w328) -> (error out=w329:errorcluster)  [unwired: 1 in, 2 out]
              }
            }
          }
          frame "Hidden", "Hide" {
            w330 = T4."Hidden" ("State")
            n147 = property class="VI"(reference=w336, error in=w335) -> (reference out=w333:refnum<vi>, error out=w334:errorcluster, "FP.State"=w332:T4)
            n148 = Not Equal?(x=w332, y=w330) -> (x != y?=w331:bool)
            n149 = case shown="True" w331 {
              tunnel: [w341 w342] -> w337
              tunnel: w334 -> [w340 w342]
              tunnel: w333 -> [w339 _]
              tunnel: w330 -> [w338 _]
              frame True {
                n150 = invoke class="VI" method="FP.Open"(reference=w339, error in=w340, "State"=w338) -> (error out=w341:errorcluster)  [unwired: 2 in, 4 out]
              }
              frame False {
              }
            }
          }
          frame "Minimize", "Minimized" {
            w343 = T4."Minimized" ("State")
            n151 = property class="VI"(reference=w349, error in=w348) -> (reference out=w346:refnum<vi>, error out=w347:errorcluster, "FP.State"=w345:T4)
            n152 = Not Equal?(x=w345, y=w343) -> (x != y?=w344:bool)
            n153 = case shown="True" w344 {
              tunnel: [w354 w355] -> w350
              tunnel: w347 -> [w353 w355]
              tunnel: w346 -> [w352 _]
              tunnel: w343 -> [w351 _]
              frame True {
                n154 = invoke class="VI" method="FP.Open"(reference=w352, error in=w353, "State"=w351) -> (error out=w354:errorcluster)  [unwired: 2 in, 4 out]
              }
              frame False {
              }
            }
          }
          frame "Maximize", "Maximized" {
            w356 = T4."Maximized" ("State")
            n155 = property class="VI"(reference=w362, error in=w361) -> (reference out=w359:refnum<vi>, error out=w360:errorcluster, "FP.State"=w358:T4)
            n156 = Not Equal?(x=w358, y=w356) -> (x != y?=w357:bool)
            n157 = case shown="True" w357 {
              tunnel: [w367 w368] -> w363
              tunnel: w360 -> [w366 w368]
              tunnel: w359 -> [w365 _]
              tunnel: w356 -> [w364 _]
              frame True {
                n158 = invoke class="VI" method="FP.Open"(reference=w365, error in=w366, "State"=w364) -> (error out=w367:errorcluster)  [unwired: 2 in, 4 out]
              }
              frame False {
              }
            }
          }
        }
        n159 = call <vilib>:"Add State(s) to Queue__JKI_lib_State_Machine.vi"("State(s) in (\"\")"=w303) -> ("States Out"=w302:string)  [unwired: 14 in]
      }
      frame "CSM: Module List Changed", "UI: Refresh CSM List" {
        n160 = control-ref of="CSM"() -> (w378:refnum<vi>)
        n161 = property on="Property Node" class="CmbBox"(reference=w378) -> (reference out=w370:refnum<vi>, "Value"=w374:string)  [unwired: 1 in, 1 out]
        n162 = call "CSM - List Modules.vi"("Scope (Normal)"="Scope") -> ("error out"=w377:errorcluster, "Module Names"=w372:string[])  [unwired: 9 in]
        n163 = Search 1D Array(1D array=w372, element=w374) -> (index of element=w376:i32)  [unwired: 1 in]
        n164 = Greater Or Equal To 0?(x=w376) -> (x >= 0?=w375:bool)
        n165 = Index Array(array=w372) -> (element=w373:string)  [unwired: 1 in]
        n166 = Select(t=w374, s=w375, f=w373) -> (s? t:f=w371:string)
        n167 = call <vilib>:"Simple Error Handler.vi"("error in (no error)"=w377) -> ()  [unwired: 4 in, 5 out]
        n168 = property on="Property Node" class="CmbBox"(reference=w370, "Strings[]"=w372, "Val(Sgnl)"=w371) -> ()  [unwired: 1 in, 2 out]
      }
      frame "UI: Try to Change Command" {
        n169 = control-ref of="CSM"() -> (w395:refnum<vi>)
        n170 = property on="Property Node" class="CmbBox"(reference=w395) -> (reference out=w385:refnum<vi>, error out=w384:errorcluster, "Strings[]"=w382:string[])  [unwired: 1 in]
        n171 = call "CSM - Convert HexStr to Data.vi"("HEX String"=w394) -> ("Variant"=w392:variant, "error out"=w393:errorcluster)  [unwired: 7 in]
        n172 = Variant To Data(error in=w393, type="", Variant=w392) -> (data=w390:string)  [unwired: 1 out]
        n173 = call "Remove Comments from Single-line.vi"("single-line text"=w390) -> ("single-line text without comments"=w389:string)  [unwired: 2 in]
        n174 = call "Split Single-line Message.vi"("single-line text"=w389) -> ("source/target"=w388:string)  [unwired: 6 in, 3 out]
        n175 = To Lower Case(string=w382) -> (all lower case string=w387:string[])
        n176 = To Lower Case(string=w388) -> (all lower case string=w386:string)
        n177 = Search 1D Array(1D array=w387, element=w386) -> (index of element=w383:i32)  [unwired: 1 in]
        n178 = case shown="Default" w383 {
          selector: w383 -> [_ w400]
          tunnel: w385 -> [_ w403]
          tunnel: w384 -> [_ w402]
          tunnel: w382 -> [_ w401]
          frame -1 {
          }
          frame Default {
            n179 = Index Array(array=w401, index=w400) -> (element=w399:string)
            n180 = property on="Property Node" class="CmbBox"(reference=w403, error in=w402, "Value"=w399) -> ()  [unwired: 2 out]
          }
        }
      }
      frame "UI: Insert LogViewer" {
        # "Replace with your own CSM Module"
        n181 = vi-ref "LogViewer.vi"() -> (w409:refnum<vi>)
        n182 = property class="VI Interface Type 0"(reference=w409) -> (reference out=w413:refnum<vi>, error out=w411:errorcluster, "Path"=w410:path)  [unwired: 1 in]
        n183 = Open VI Reference(type specifier VI Refnum (for type only)=w413, vi path=w410, options=128, error in (no error)=w411) -> (vi reference=w412:refnum<vi>, error out=w408:errorcluster)  [unwired: 2 in]
        n184 = call "Concatenate Submodule Name.vi"("Module Name"="logviewer", "Group Name"=w405) -> ("Submodule Name"=w406:string)  [unwired: 9 in]
        n185 = call-by-ref "Start Asynchronous Call"(reference=w412, error in=w408, "Current Module(\"\" to generate an ID)"=w406) -> (reference out=w407:refnum<vi>, error out=w414:errorcluster)  [unwired: 11 in]
        n186 = invoke on="subpnl" class="SubPnl" method="Insert VI"("VI Ref"=w407) -> ()  [unwired: 3 in, 4 out]
        n187 = Close Reference(reference=w407, error in (no error)=w414) -> ()  [unwired: 1 out]
      }
      frame "UI: Insert History View" {
        n188 = vi-ref "DebugConsole.lvlib:HistoryList.vi"() -> (w425:refnum<vi>)
        n189 = property class="VI Interface Type 0"(reference=w425) -> (reference out=w429:refnum<vi>, error out=w427:errorcluster, "Path"=w426:path)  [unwired: 1 in]
        n190 = Open VI Reference(type specifier VI Refnum (for type only)=w429, vi path=w426, options=128, error in (no error)=w427) -> (vi reference=w428:refnum<vi>, error out=w424:errorcluster)  [unwired: 2 in]
        n191 = call "Concatenate Submodule Name.vi"("Module Name"="historyView", "Group Name"=w421) -> ("Submodule Name"=w422:string)  [unwired: 9 in]
        n192 = call-by-ref "Start Asynchronous Call"(reference=w428, error in=w424, "Current Module(\"\" to generate an ID)"=w422) -> (reference out=w423:refnum<vi>, error out=w430:errorcluster)  [unwired: 11 in]
        n193 = control-ref of="subpnl"() -> (w419:refnum<vi>)
        n194 = invoke on="Invoke Node" class="SubPnl" method="Insert VI"(reference=w419, "VI Ref"=w423) -> ()  [unwired: 2 in, 4 out]
        n195 = Close Reference(reference=w423, error in (no error)=w430) -> ()  [unwired: 1 out]
      }
      frame "UI: Insert Console" {
        n196 = Unbundle By Name(w438) -> ("ConsoleUI"=w437:refnum<vi>[])
        n197 = Index Array(array=w437, index="Console") -> (element=w435:refnum<vi>)
        n198 = control-ref of="subpnl"() -> (w439:refnum<vi>)
        n199 = invoke on="Invoke Node" class="SubPnl" method="Insert VI"(reference=w439, "VI Ref"=w435) -> ()  [unwired: 2 in, 4 out]
      }
      frame "UI: Refresh UI" {
      }
      frame "---------- Macro ----------" {
        # "Do not put any code in this frame.\n(It is a separator no-op. You can make a copy of this frame to create a new Macro frame)"
        n200 = call <vilib>:"Add State(s) to Queue__JKI_lib_State_Machine.vi"("State(s) in (\"\")"=w448) -> ("States Out"=w447:string)  [unwired: 14 in]
      }
      frame "Macro: Initialize" {
        # "Initialization Macro\n(This is called once, when the VI starts)"
        n201 = call <vilib>:"Add State(s) to Queue__JKI_lib_State_Machine.vi"("State(s) in Front (\"\")"="Data: Initialize\nData: Initialize References\nInitialize Core Data\nUI: Initialize\nData: Load Arguments Config File\nUI: Front Panel State >> Open\nAction: Start Message Console\nAction: Start Broadcast Console\nAction: Start Registration Console\nAction: Start Scripts Console\nAction: Start Information Console\nUI: Insert History View\nUI: Insert LogViewer\nUI: Insert Console\nUI: Refresh CSM List\nUI: Refresh UI\nAction: Change Btn States", "State(s) in (\"\")"=w453) -> ("States Out"=w452:string)  [unwired: 13 in]
      }
      frame "Macro: Exit" {
        # "Exit Macro\n(This is called once, when the VI exits)"
        n202 = Concatenate Strings(w454, ".*") -> (w455:string)
        n203 = call "_Broadcast Message.vi"("Module Pattern (support *)"=w455, "Broadcast"=_BroadcastDef."Macro: Exit") -> ("Error out"=w456:errorcluster)  [unwired: 9 in]
        n204 = disable-structure shown="Disabled" {
          disable-tunnel: w456 -> [w467 _]
          disable-tunnel: w454 -> [w465 _]
          frame Disabled {
            n205 = Get Date/Time In Seconds() -> (seconds since 1Jan1904=w466:timestamp)
            n206 = while {
              tunnel: w467 -> [w481]
              tunnel: w465 -> [w480]
              tunnel: w466 -> [w473]
              stop <- w470 stop-if-true
              n207 = call "_Engine.vi"("Enum"=_action."List", "Error in"=w481) -> ("Array"=w478:string[])  [unwired: 7 in, 2 out]
              n208 = Get Date/Time In Seconds() -> (seconds since 1Jan1904=w474:timestamp)
              n209 = Search 1D Array(1D array=w478, element=w480) -> (index of element=w479:i32)  [unwired: 1 in]
              n210 = Subtract(x=w474, y=w473) -> (x-y=w472:dbl)
              n211 = Delete From Array(array=w478, index=w479) -> (array with subset deleted=w477:string[])  [unwired: 1 in, 1 out]
              n212 = Greater?(x=w472, y=5.0) -> (0:w468:bool)
              n213 = Empty Array?(array=w477) -> (empty?=w469:bool)
              n214 = Wait (ms)(milliseconds to wait=u32 10) -> ()  [unwired: 1 out]
              n215 = Or(x=w469, y=w468) -> (x .or. y?=w470:bool)
            }
          }
          frame Enabled {
          }
        }
        n216 = call <vilib>:"Add State(s) to Queue__JKI_lib_State_Machine.vi"("State(s) at Back (\"\")"="Data: Save Arguments Config File\nData: Cleanup\nExit") -> ("States Out"=w459:string)  [unwired: 14 in]
        n217 = call <vilib>:"Add State(s) to Queue__JKI_lib_State_Machine.vi"("State(s) in Front (\"\")"=w459, "State(s) in (\"\")"=w464) -> ("States Out"=w463:string)  [unwired: 13 in]
      }
      frame "---------- Action ----------" {
        # "Template Separator\n(You can make a copy of, or modify, this frame)"
        n218 = call <vilib>:"Add State(s) to Queue__JKI_lib_State_Machine.vi"("State(s) in (\"\")"=w485) -> ("States Out"=w484:string)  [unwired: 14 in]
      }
      frame "Action: Change Btn States" {
        n219 = local read "CSM"() -> (w489:string)
        n220 = case shown="Default" w489 {
          selector: w489 -> [_ w493]
          tunnel: w488 -> [_ w506]
          frame "" {
          }
          frame Default {
            n221 = call "CSM - Module VI Reference.vi"("Response Timeout (-2 Using Global Settings)"=1000 ("Response Timeout(5000 ms)"), "Current Module (\"\" to Generate an ID)"=w506, "CSM Name"=w493) -> ("error out"=w503:errorcluster, "CSM Module VIRef"=w504:refnum<vi>)  [unwired: 7 in]
            n222 = property class="VI"(reference=w504, error in=w503) -> (reference out=w497:refnum<vi>, "IsInPackedLibrary"=→"inlvlibp":bool, "Diagram"=w496:refnum<vi>)  [unwired: 1 out]
            n223 = Close Reference(reference=w496) -> (error out=w495:errorcluster)  [unwired: 1 in]
            n224 = call <vilib>:"Clear Errors.vi"("error in (no error)"=w495) -> ("error out"=w494:errorcluster)  [unwired: 5 in, 1 out]
            n225 = Close Reference(reference=w497, error in (no error)=w494) -> ()  [unwired: 1 out]
            n226 = Not A Number/Path/Refnum?(number/path/refnum=w496) -> (NaN/Path/Refnum?=w500:bool)
            n227 = Select(t=2, s=w500, f=0) -> (s? t:f=w501:i32)
            n228 = property on="Toolbar.Open BD" class="Bool"("DisabledEnum"=w501) -> ()  [unwired: 2 in, 2 out]
          }
        }
        n229 = local read "CSM"() -> (w487:string)
        n230 = call "_Broadcast Message.vi"("Argument(\"\")"=w487, "Broadcast"=_BroadcastDef."CSM: Module Selected") -> ()  [unwired: 9 in, 1 out]
      }
      frame "No Peroidic Log over 1s" {
        n231 = call "CSM - Generate User Global Log.vi"("Place (\"\" to Use VI's Name)"=w507, "Log"="No Peroidic Log over 1s.") -> ()  [unwired: 9 in, 1 out]
      }
      frame "Action: Start Message Console" {
        n232 = in-place {
          in-place-border: w512 -> [w518]
          # "Replace with your own CSM Module"
          n233 = in-place-cluster #1(w514) -> ("ConsoleUI"=w522:refnum<vi>[])
          n234 = vi-ref "Message Console.vi"() -> (w525:refnum<vi>)
          n235 = property class="VI Interface Type 0"(reference=w525) -> (reference out=w529:refnum<vi>, error out=w527:errorcluster, "Path"=w526:path)  [unwired: 1 in]
          n236 = Open VI Reference(type specifier VI Refnum (for type only)=w529, vi path=w526, options=128, error in (no error)=w527) -> (vi reference=w528:refnum<vi>, error out=w524:errorcluster)  [unwired: 2 in]
          n237 = call "Concatenate Submodule Name.vi"("Module Name"="MsgConsole", "Group Name"=w518) -> ("Submodule Name"=w517:string)  [unwired: 9 in]
          n238 = call-by-ref "Start Asynchronous Call"(reference=w528, error in=w524, "Name"=w517) -> (reference out=w520:refnum<vi>, error out=w530:errorcluster)  [unwired: 11 in]
          n239 = Close Reference(reference=w520, error in (no error)=w530) -> ()  [unwired: 1 out]
          n240 = Build Array (concatenate)(w522, w520) -> (w521:refnum<vi>[])
          n241 = in-place-cluster #1("ConsoleUI"=w521) -> (w513:T9)
        }
      }
      frame "Action: Start Broadcast Console" {
        n242 = in-place {
          in-place-border: w531 -> [w537]
          # "Replace with your own CSM Module"
          n243 = in-place-cluster #2(w533) -> ("ConsoleUI"=w541:refnum<vi>[])
          n244 = vi-ref "Broadcast Console.vi"() -> (w544:refnum<vi>)
          n245 = property class="VI Interface Type 0"(reference=w544) -> (reference out=w548:refnum<vi>, error out=w546:errorcluster, "Path"=w545:path)  [unwired: 1 in]
          n246 = Open VI Reference(type specifier VI Refnum (for type only)=w548, vi path=w545, options=128, error in (no error)=w546) -> (vi reference=w547:refnum<vi>, error out=w543:errorcluster)  [unwired: 2 in]
          n247 = call "Concatenate Submodule Name.vi"("Module Name"="BroadcastConsole", "Group Name"=w537) -> ("Submodule Name"=w536:string)  [unwired: 9 in]
          n248 = call-by-ref "Start Asynchronous Call"(reference=w547, error in=w543, "name"=w536) -> (reference out=w539:refnum<vi>, error out=w549:errorcluster)  [unwired: 11 in]
          n249 = Close Reference(reference=w539, error in (no error)=w549) -> ()  [unwired: 1 out]
          n250 = Build Array (concatenate)(w541, w539) -> (w540:refnum<vi>[])
          n251 = in-place-cluster #2("ConsoleUI"=w540) -> (w532:T9)
        }
      }
      frame "Action: Start Registration Console" {
        n252 = in-place {
          in-place-border: w550 -> [w556]
          # "Replace with your own CSM Module"
          n253 = in-place-cluster #3(w552) -> ("ConsoleUI"=w561:refnum<vi>[])
          n254 = vi-ref "Registration Console.vi"() -> (w558:refnum<vi>)
          n255 = property class="VI Interface Type 0"(reference=w558) -> (reference out=w567:refnum<vi>, error out=w565:errorcluster, "Path"=w564:path)  [unwired: 1 in]
          n256 = Open VI Reference(type specifier VI Refnum (for type only)=w567, vi path=w564, options=128, error in (no error)=w565) -> (vi reference=w566:refnum<vi>, error out=w563:errorcluster)  [unwired: 2 in]
          n257 = call "Concatenate Submodule Name.vi"("Module Name"="RegConsole", "Group Name"=w556) -> ("Submodule Name"=w557:string)  [unwired: 9 in]
          n258 = call-by-ref "Start Asynchronous Call"(reference=w566, error in=w563, "name"=w557) -> (reference out=w559:refnum<vi>, error out=w568:errorcluster)  [unwired: 11 in]
          n259 = Close Reference(reference=w559, error in (no error)=w568) -> ()  [unwired: 1 out]
          n260 = Build Array (concatenate)(w561, w559) -> (w560:refnum<vi>[])
          n261 = in-place-cluster #3("ConsoleUI"=w560) -> (w551:T9)
        }
      }
      frame "Action: Start Scripts Console" {
        n262 = in-place {
          in-place-border: w569 -> [w575]
          # "Replace with your own CSM Module"
          n263 = in-place-cluster #4(w571) -> ("ConsoleUI"=w580:refnum<vi>[])
          n264 = vi-ref "DebugConsole.lvlib:Script-Window.vi"() -> (w577:refnum<vi>)
          n265 = property class="VI Interface Type 0"(reference=w577) -> (reference out=w586:refnum<vi>, error out=w584:errorcluster, "Path"=w583:path)  [unwired: 1 in]
          n266 = Open VI Reference(type specifier VI Refnum (for type only)=w586, vi path=w583, options=128, error in (no error)=w584) -> (vi reference=w585:refnum<vi>, error out=w582:errorcluster)  [unwired: 2 in]
          n267 = call "Concatenate Submodule Name.vi"("Module Name"="ScriptConsole", "Group Name"=w575) -> ("Submodule Name"=w576:string)  [unwired: 9 in]
          n268 = call-by-ref "Start Asynchronous Call"(reference=w585, error in=w582, "name"=w576) -> (reference out=w578:refnum<vi>, error out=w587:errorcluster)  [unwired: 11 in]
          n269 = Close Reference(reference=w578, error in (no error)=w587) -> ()  [unwired: 1 out]
          n270 = Build Array (concatenate)(w580, w578) -> (w579:refnum<vi>[])
          n271 = in-place-cluster #4("ConsoleUI"=w579) -> (w570:T9)
        }
      }
      frame "Action: Start Information Console" {
        n272 = in-place {
          in-place-border: w588 -> [w594]
          n273 = in-place-cluster #5(w590) -> ("ConsoleUI"=w599:refnum<vi>[])
          n274 = vi-ref "DebugConsole.lvlib:Module Information.vi"() -> (w596:refnum<vi>)
          n275 = property class="VI Interface Type 0"(reference=w596) -> (reference out=w605:refnum<vi>, error out=w603:errorcluster, "Path"=w602:path)  [unwired: 1 in]
          n276 = Open VI Reference(type specifier VI Refnum (for type only)=w605, vi path=w602, options=128, error in (no error)=w603) -> (vi reference=w604:refnum<vi>, error out=w601:errorcluster)  [unwired: 2 in]
          n277 = call "Concatenate Submodule Name.vi"("Module Name"="ModuleInfo", "Group Name"=w594) -> ("Submodule Name"=w595:string)  [unwired: 9 in]
          n278 = call-by-ref "Start Asynchronous Call"(reference=w604, error in=w601, "name"=w595) -> (reference out=w597:refnum<vi>, error out=w606:errorcluster)  [unwired: 11 in]
          n279 = Close Reference(reference=w597, error in (no error)=w606) -> ()  [unwired: 1 out]
          n280 = Build Array (concatenate)(w599, w597) -> (w598:refnum<vi>[])
          n281 = in-place-cluster #5("ConsoleUI"=w598) -> (w589:T9)
        }
      }
    }
  }
  n282 = disable-structure shown="Disabled" {
    frame Disabled {
      n283 = case shown="\"Module Created\", \"Module Destroyed\"" {
        selector: _ -> [_ _]
        tunnel: _ -> [_ w608]
        frame "User Log", Default {
        }
        frame "Module Created", "Module Destroyed" {
          n284 = Generate User Event(user event=w608, event data cluster="UI: Refresh CSM List" ("State(s) in Front (\"\")")) -> ()  [unwired: 2 in, 2 out]
        }
      }
    }
    frame Enabled {
    }
  }
  n285 = control-ref of="Current VI Reference"() -> (w3:refnum<vi>)
  n286 = call "Close FP if in LabVIEW Dir.vi"("VI Refnum"=w3, "Error in"=w2) -> ("Error out"=w4:errorcluster)  [unwired: 9 in]
  n287 = call <vilib>:"Clear Errors.vi"("error in (no error)"=w4) -> ()  [unwired: 5 in, 2 out]
